vi "Wait For Previous.vi"(8 "error in (no error)":errorcluster, 9 "timeout in ms (0)":i32 format="%d ms", 11 "Transfer Group in":refnum<class "Transfer Group.lvclass">) -> (0 "error out":errorcluster, 1 "move data":bool, 2 "ready":bool, 3 "Transfer Group out":refnum<class "Transfer Group.lvclass">)   [LabVIEW 2020, in "DSF Core.lvlib" / "Transfer Group.lvclass"]
uses:
  Transfer Group.lvclass
  Typedefs/DSF Direction.ctl
  DSF Core.lvlib
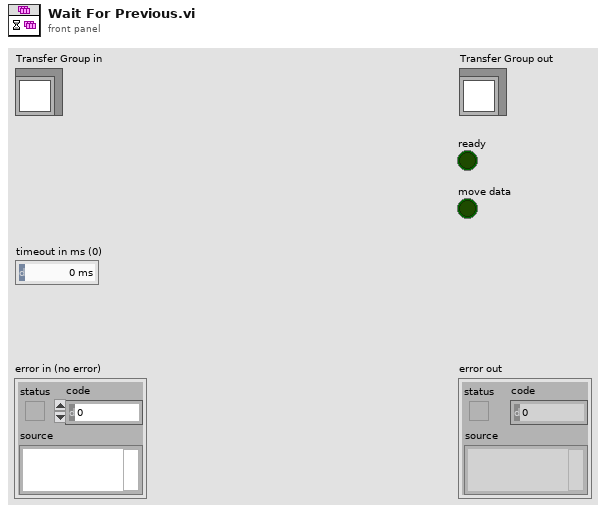
[diagram p1: front panel]
types:
  T1 = typedef "DSF Core.lvlib/DSF Direction.ctl" = enum8{"Tx", "Rx"}
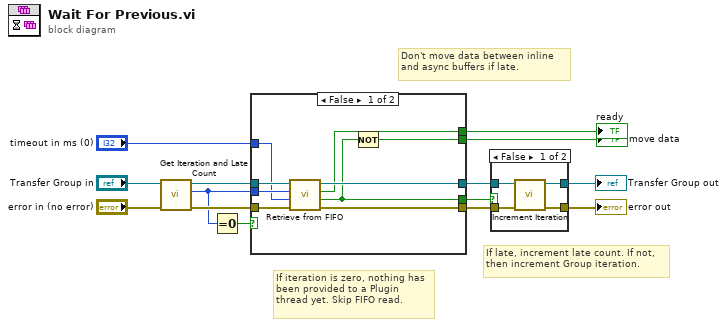
[diagram p0: block diagram]
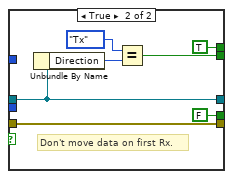
[diagram p2: hidden frame]
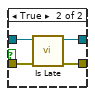
[diagram p3: hidden frame]
diagram:
  # "Don't move data between inline and async buffers if late."
  # "If late, increment late count. If not, then increment Group iteration."
  # "If iteration is zero, nothing has been provided to a Plugin thread yet. Skip FIFO read."
  n1 = call "Get Iteration and Late Count.vi"("error in (no error)"="error in (no error)", "Transfer Group in"="Transfer Group in") -> ("error out"=w13:errorcluster, "iteration"=w12:u64, "Transfer Group out"=w11:refnum<class "Transfer Group.lvclass">)  [unwired: 6 in, 1 out]
  n2 = Equal To 0?(x=w12) -> (x = 0?=w14:bool)
  n3 = case shown="False" w14 {
    tunnel: w13 -> [w23 w30]
    tunnel: [w18 w26] -> w5
    tunnel: [w16 w30] -> w4
    tunnel: w11 -> [w22 w26]
    tunnel: w12 -> [w21 _]
    tunnel: [w17 TRUE ("iteration valid?")] -> w8
    tunnel: "timeout in ms (0)" -> [w20 _]
    tunnel: [w19 w25] -> w6
    tunnel: [w15 FALSE ("late")] -> w1
    frame False {
      n4 = call "Retrieve from FIFO.vi"("error in (no error)"=w23, "timeout in ms (0)"=w20, "expected iteration"=w21, "Transfer Group in"=w22) -> ("error out"=w16:errorcluster, "late"=w15:bool, "ready"=w17:bool, "Transfer Group out"=w18:refnum<class "Transfer Group.lvclass">)  [unwired: 4 in]
      n5 = Not(x=w15) -> (.not. x?=w19:bool)
    }
    frame True {
      # "Don't move data on first Rx."
      n6 = Unbundle By Name(w26) -> ("Direction"=w28:T1)
      n7 = Equal?(x=DSF_Direction."Tx" ("y"), y=w28) -> (x = y?=w25:bool)
    }
  }
  "ready" <- w8
  "move data" <- w6
  n8 = case shown="False" w1 {
    tunnel: w5 -> [w34 w38]
    tunnel: w4 -> [w33 w37]
    tunnel: [w32 w36] -> w3
    tunnel: [w31 w35] -> w2
    frame False {
      n9 = call "Increment Iteration.vi"("error in (no error)"=w33, "Transfer Group in"=w34) -> ("error out"=w31:errorcluster, "Transfer Group out"=w32:refnum<class "Transfer Group.lvclass">)  [unwired: 8 in]
    }
    frame True {
      n10 = call "Is Late.vi"("error in (no error)"=w37, "Transfer Group in"=w38) -> ("error out"=w35:errorcluster, "Transfer Group out"=w36:refnum<class "Transfer Group.lvclass">)  [unwired: 8 in]
    }
  }
  "error out" <- w2
  "Transfer Group out" <- w3
